vi "Erase Stream Buffer.vi"(8 "error in (no error)":errorcluster, 9 "Device Number":string, 10 "Buffer Number (1)":u8=1, 11 "VISA resource name":refnum<visa-resource-name>) -> (0 "error out":errorcluster, 3 "VISA resource name out":refnum<visa-resource-name>)   [LabVIEW 2018, in "Zaber A Series.lvlib"]
doc: "Erases a buffered stream, removing it from device memory. It is best practice to do this before opening a stream to add new commands. The input buffer number must be between 1 and the value of the \"stream.numbufs\" setting on the device - use the Get Stream Support Info VI to get this value. Note this is the same as the Buffer Number input to the Open Stream VI, not the Stream Number input.\n\nThe erase operation only applies to streams that have been saved in buffers; it does not work on live streams.\n\nThis VI does not check in advance for error conditions such as streams not being supported.\n\nThis VI requires that the Initialize VI has been called with the same serial port."
uses:
  Zaber A Series.lvlib
  Private/All Commands.ctl
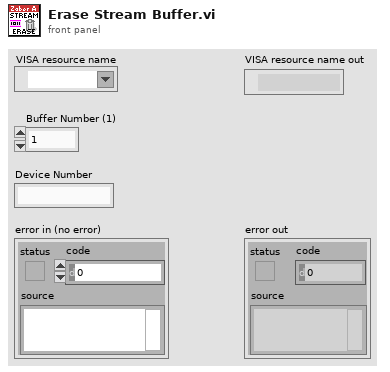
[diagram p1: front panel]
types:
  T1 = typedef "Zaber A Series.lvlib/All Commands.ctl" = string
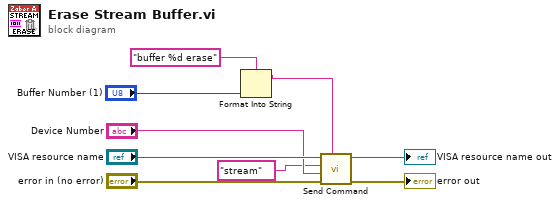
[diagram p0: block diagram]
diagram:
  n1 = Format Into String(format string="buffer %d erase", "Buffer Number (1)") -> (resulting string=w4:string)  [unwired: 2 in, 1 out]
  n2 = call "Send Command.vi"("Data"=w4, "error in (no error)"="error in (no error)", "Device and Axis"="Device Number", "Command"=T1 "stream" ("Complete Command List"), "VISA resource name"="VISA resource name") -> ("error out"=→"error out":errorcluster, "VISA resource name out"=→"VISA resource name out":refnum<visa-resource-name>)  [unwired: 1 in, 4 out]
